vi "BlenderMain.vi"(8 "error in (no error)":errorcluster, 9 "Reverse":bool, 10 "Forward":bool, 11 "Control Mode":enum16{"Open", "Control"}(ring)) -> (0 "error out":errorcluster)   [LabVIEW 2016]
uses:
  <vilib>/Rock Robotics/SystemInterfaces/DIO/FPGA_DIORelayChannel.ctl
  <vilib>/Rock Robotics/WPI/Relay/WPI_RelayValue.ctl
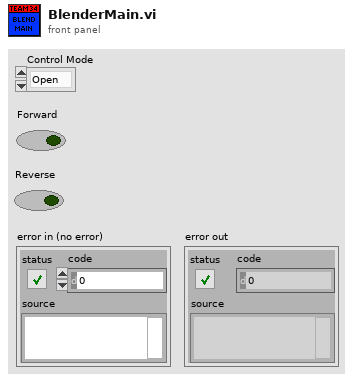
[diagram p1: front panel]
types:
  T1 = typedef "FPGA_DIORelayChannel.ctl" = enum8{"Relay 0", "Relay 1", "Relay 2", "Relay 3", "Invalid"}
  T2 = typedef "WPI_RelayValue.ctl" = enum16{"Off", "On", "Forward", "Reverse"}
  T3 = typedef "WPI_RelayDevRef.ctl" = cluster{"DevStatus":errorcluster, "Relay Channel":T1, "Relay Direction":T4}
  T4 = typedef "WPI_RelayDirection.ctl" = enum16{"Both directions", "Forward only", "Reverse only"}
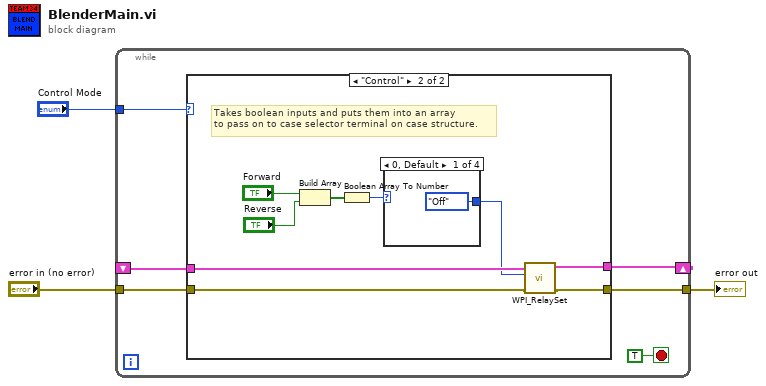
[diagram p0: block diagram]
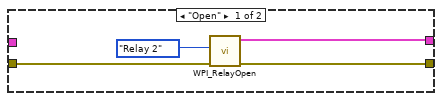
[diagram p2: hidden frame]
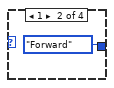
[diagram p3: hidden frame]
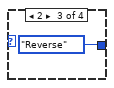
[diagram p4: hidden frame]
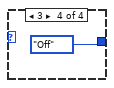
[diagram p5: hidden frame]
diagram:
  n1 = while {
    tunnel: "Control Mode" -> [w8]
    tunnel: "error in (no error)" -> [w7]
    tunnel: [w6] -> w3
    shift-right: [w5] -> _
    shift-left: _ -> [w4]
    stop <- TRUE stop-if-true
    n2 = case shown="\"Control\"" w8 {
      tunnel: w7 -> [w13 w15]
      tunnel: [w12 w16] -> w6
      tunnel: [w10 w17] -> w5
      tunnel: w4 -> [_ w18]
      frame "Open" {
        n3 = call <vilib>:"WPI_RelayOpen.vi"("error in (no error)"=w13, "Relay Channel"=FPGA_DIORelayChannel."Relay 2") -> ("error out"=w12:errorcluster, "RelayDevRef"=w10:T3)  [unwired: 8 in]
      }
      frame "Control" {
        # "Takes boolean inputs and puts them into an array\nto pass on to case selector terminal on case structure."
        n4 = Build Array("Forward", "Reverse") -> (w20:bool[])
        n5 = Boolean Array To Number(Boolean array=w20) -> (number=w19:u32)
        n6 = case shown="0, Default" w19 {
          tunnel: [WPI_RelayValue."Off" ("RelayValue") WPI_RelayValue."Forward" ("RelayValue") WPI_RelayValue."Reverse" ("RelayValue") WPI_RelayValue."Off" ("RelayValue")] -> w14
          frame 0, Default {
          }
          frame 1 {
          }
          frame 2 {
          }
          frame 3 {
          }
        }
        n7 = call <vilib>:"WPI_RelaySet.vi"("error in (no error)"=w15, "RelayValue"=w14, "RelayDevRef"=w18) -> ("error out"=w16:errorcluster, "RelayDevRef"=w17:T3)  [unwired: 7 in]
      }
    }
  }
  "error out" <- w3
